vi "文件夹有效性.vi"(9 "路径":string, 11 "配置":string) -> (1 "路径":path, 3 "Valid":bool)   [LabVIEW 2015]
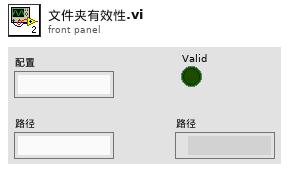
[diagram p1: front panel]
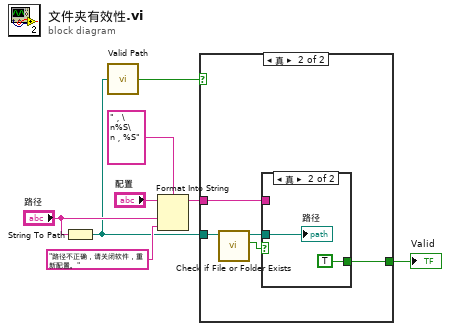
[diagram p0: block diagram]
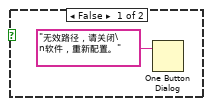
[diagram p2: hidden frame]
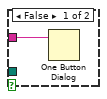
[diagram p3: hidden frame]
diagram:
  n1 = String To Path(string="路径") -> (path=w2:path)
  n2 = call "Valid Path.vi"("Path"=w2) -> ("Valid"=w3:bool)
  n3 = Format Into String(format string="，\n%S\n，%S" ("格式字符串"), initial string="配置", "路径", "路径不正确，请关闭软件，重新配置。") -> (resulting string=w8:string)  [unwired: 1 in, 1 out]
  n4 = case shown="真" w3 {
    tunnel: w8 -> [_ w14]
    tunnel: w2 -> [_ w11]
    tunnel: [_ w10] -> w1
    frame False {
      n5 = One Button Dialog(message="无效路径，请关闭\n软件，重新配置。") -> ()  [unwired: 1 in, 1 out]
    }
    frame True {
      n6 = call <vilib>:"Check if File or Folder Exists.vi"("path"=w11) -> ("file or folder exists?"=w12:bool, "dup path"=w13:path)  [unwired: 8 in, 1 out]
      n7 = case shown="真" w12 {
        tunnel: w13 -> [_ w17]
        tunnel: w14 -> [w15 _]
        tunnel: [_ TRUE] -> w10
        frame False {
          n8 = One Button Dialog(message=w15) -> ()  [unwired: 1 in, 1 out]
        }
        frame True {
          "路径" <- w17
        }
      }
    }
  }
  "Valid" <- w1
